vi "qp_find initial feasible solution.vi"(6 "tolerance":dbl=1e-05, 8 "error in (no error)":errorcluster, 11 "qp data in":T1) -> (0 "error out":errorcluster, 3 "qp data in":T1)   [LabVIEW 2014, in "NI_Gmath.lvlib"]
uses:
  NI_Gmath.lvlib
  qp_problem data.ctl
  A x Vector.vi
  Real A x B.vi
  Real Dot Product.vi
  Create Special Real Matrix.vi
  ones_1d.vi
  zeroes_1d.vi
  zeroes_2d.vi
  Matrix left divisionMM.vi
  NI_AALBase.lvlib
  NI_AALPro.lvlib
panel:
  out "Numeric":i32
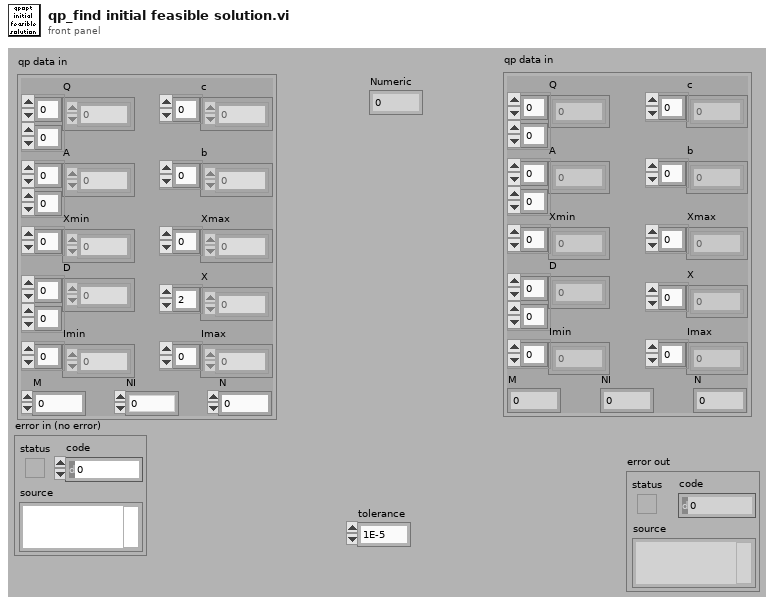
[diagram p1: front panel]
types:
  T1 = typedef "NI_Gmath.lvlib/qp_problem data.ctl" = cluster{"Q":dbl[][], "c":dbl[], "A":dbl[][], "b":dbl[], "Xmin":dbl[], "Xmax":dbl[], "M":i32, "N":i32, "D":dbl[][], "Imax":dbl[], "Imin":dbl[], "NI":i32, "X":dbl[]}
  T2 = enum32{"Identity", "Diagonal", "Toepliz", "Vandermonde", "Companion"}
  T3 = typedef "NI_Matrix.lvlib/RealMatrix.ctl" = dbl[][]
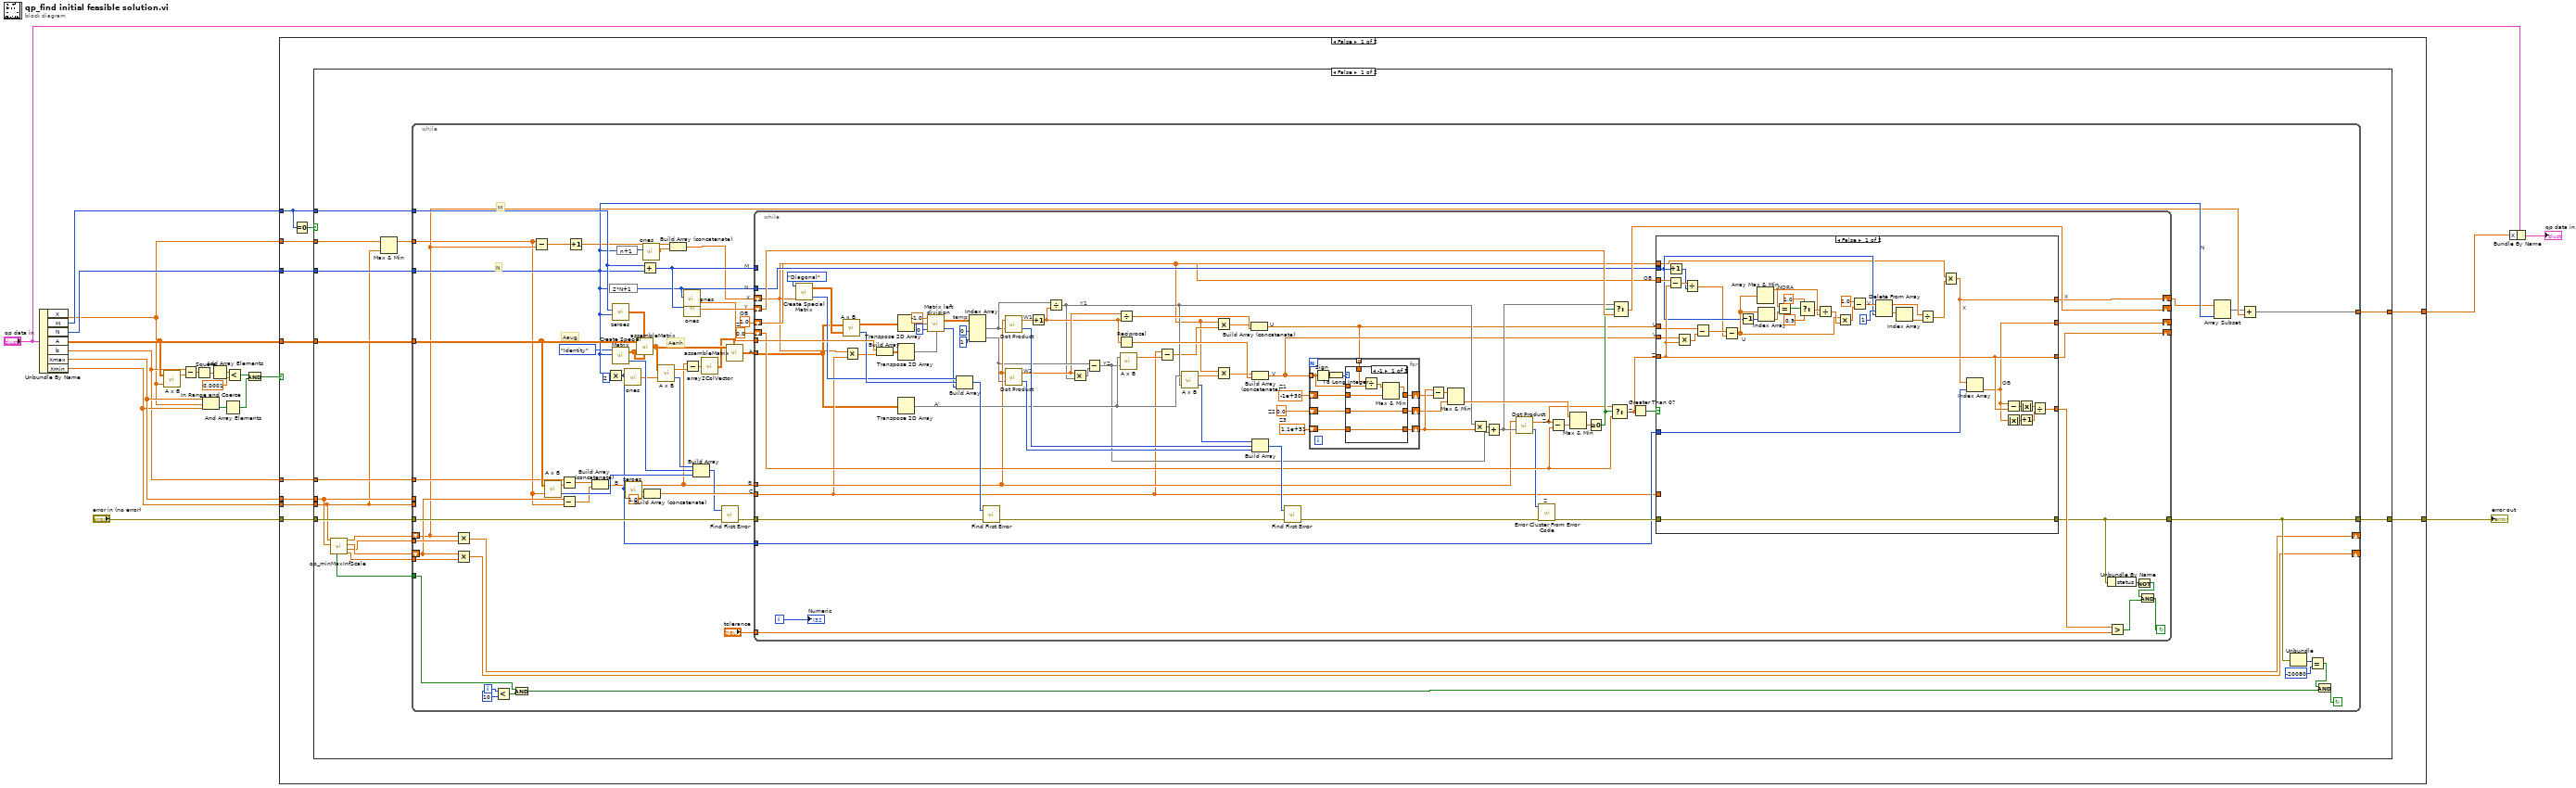
[diagram p0: block diagram]
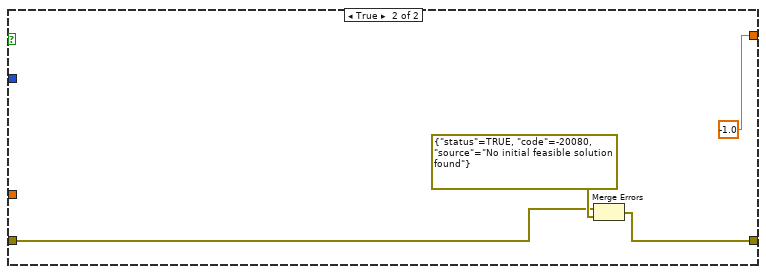
[diagram p2: hidden frame]
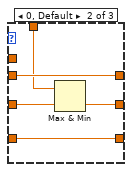
[diagram p3: hidden frame]
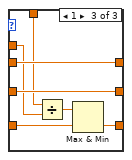
[diagram p4: hidden frame]
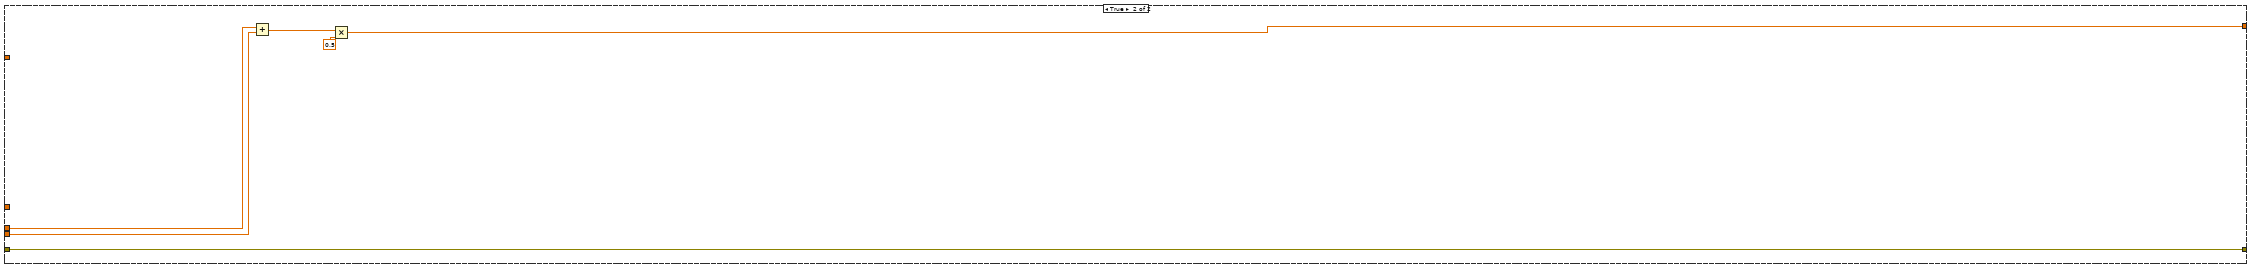
[diagram p5: hidden frame]
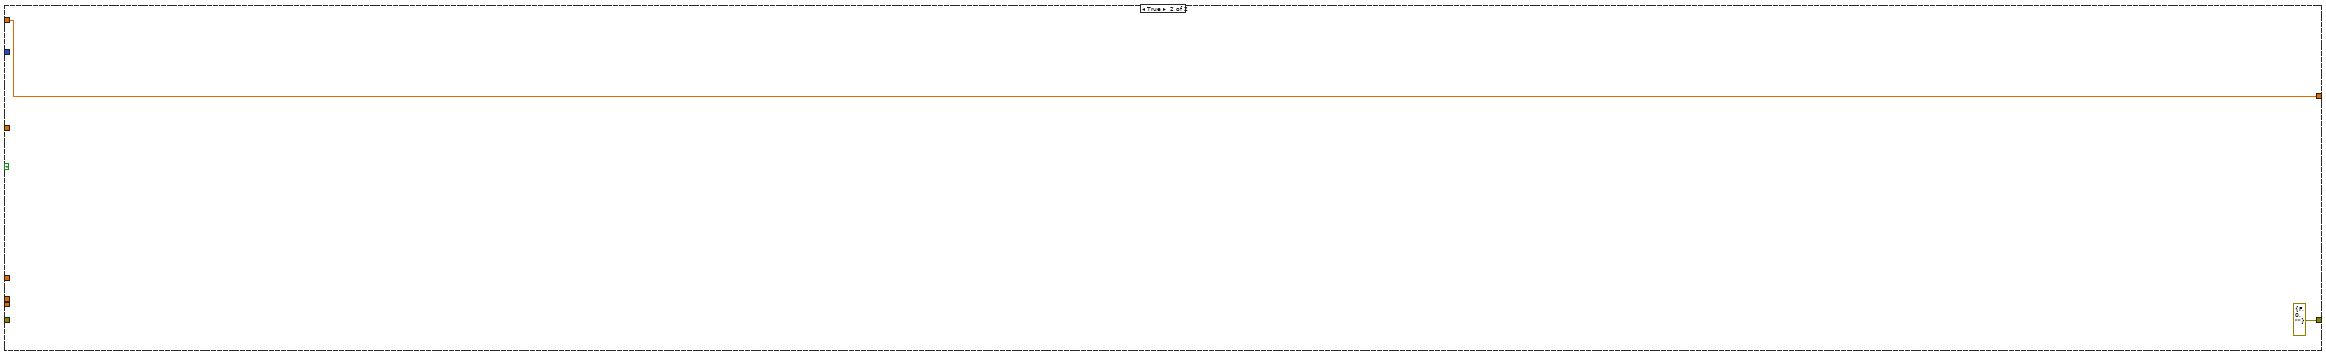
[diagram p6: hidden frame]
diagram:
  n1 = Unbundle By Name("qp data in") -> ("X"=w4:dbl[], "M"=w20:i32, "N"=w21:i32, "A"=w7:dbl[][], "b"=w6:dbl[], "Xmax"=w9:dbl[], "Xmin"=w8:dbl[])
  n2 = call-poly "A x B.vi"("Vector"=w4, "A"=w7) -> ("A x Vector"=w17:dbl[])  [unwired: 1 out]
  n3 = Subtract ("Subtract.vi")(x=w6, y=w17) -> (x-y=w16:dbl[])
  n4 = Square(x=w16) -> (x^2=w15:dbl[])
  n5 = In Range and Coerce(upper limit=w9, x=w4, lower limit=w8) -> (In Range?=w11:bool[])  [unwired: 1 out]
  n6 = Add Array Elements(numeric array=w15) -> (sum=w14:dbl)
  n7 = And Array Elements(Boolean array=w11) -> (logical AND=w10:bool)
  n8 = Less?(x=w14, y=0.0001) -> (x < y?=w12:bool)
  n9 = And(x=w12, y=w10) -> (x .and. y?=w5:bool)
  n10 = case shown="False" w5 {
    tunnel: w21 -> [w32 _]
    tunnel: w20 -> [w30 _]
    tunnel: [w29 errorcluster {"status"=FALSE, "code"=0, "source"=""} ("error in (no error)")] -> w19
    tunnel: "error in (no error)" -> [w28 _]
    tunnel: [w27 w267] -> w2
    tunnel: w4 -> [w26 w267]
    tunnel: w9 -> [w25 _]
    tunnel: w8 -> [w24 _]
    tunnel: w7 -> [w23 _]
    tunnel: w6 -> [w22 _]
    frame False {
      n11 = Equal To 0?(x=w30) -> (x = 0?=w31:bool)
      n12 = case shown="False" w31 {
        tunnel: [w47 w261] -> w27
        tunnel: w32 -> [w36 _]
        tunnel: w23 -> [w43 _]
        tunnel: w22 -> [w48 _]
        tunnel: w30 -> [w44 _]
        tunnel: [w46 w260] -> w29
        tunnel: w28 -> [w45 w260]
        tunnel: w24 -> [w35 w264]
        tunnel: w25 -> [w37 w265]
        tunnel: w26 -> [w33 _]
        frame False {
          n13 = call "qp_minMaxInfScale.vi"("Xmax"=w37, "Xmin"=w35) -> ("Xmax scale"=w39:dbl[], "Xmin scale"=w40:dbl[], "Xmax"=w41:dbl[], "Xmin"=w42:dbl[], "loop?"=w38:bool)  [unwired: 2 in]
          n14 = Max & Min(x=w33, y=w35) -> (max(x,y)=w34:dbl[])  [unwired: 1 out]
          n15 = while {
            tunnel: w48 -> [w90]
            tunnel: [w49] -> w47
            tunnel: [w96] -> w46
            tunnel: w45 -> [w108]
            tunnel: w44 -> [w107]
            tunnel: w43 -> [w106]
            tunnel: w36 -> [w105]
            tunnel: w34 -> [w51]
            shift-right: [w92] -> _
            shift-left: w42 -> [w88]
            shift-right: [w91] -> _
            shift-left: w41 -> [w89]
            tunnel: w40 -> [w94]
            tunnel: w39 -> [w93]
            tunnel: w38 -> [w101]
            tunnel: w37 -> [_]
            tunnel: w35 -> [_]
            i -> [w104]
            stop <- w100 continue-if-true
            w78 = 0.0  # Z
            w79 = 1.0  # OB
            # "Aaug"
            # "Aenh"
            # "M"
            # "N"
            # "N"
            # "Y"
            # "X"
            # "C"
            # "N"
            # "M"
            # "B"
            # "A"
            # "B"
            n16 = Multiply(x=w88, y=w94) -> (x*y=w92:dbl[])
            n17 = Multiply(x=w89, y=w93) -> (x*y=w91:dbl[])
            n18 = Less?(x=w104, y=10) -> (x < y?=w102:bool)
            n19 = And(x=w101, y=w102) -> (x .and. y?=w99:bool)
            n20 = Subtract(x=w51, y=w88) -> (x-y=w62:dbl[])
            n21 = call-poly "A x B.vi"("Vector"=w51, "A"=w106) -> ("error"=w87:i32, "A x Vector"=w84:dbl[])
            n22 = Subtract(x=w90, y=w84) -> (x-y=w63:dbl[])
            n23 = Subtract(x=w89, y=w51) -> (x-y=w60:dbl[])
            n24 = Increment(x=w62) -> (x+1=w61:dbl[])
            n25 = Build Array (concatenate)(w63, w60) -> (w56:dbl[])
            n26 = Multiply(x=w105, y=2) -> (x*y=w59:i32)
            n27 = expression code="2*N+1"(w105) -> (w52:i32)
            n28 = call-poly "zeroes.vi"("m"=w107, "n"=w105) -> ("ones"=w76:dbl[][])  [unwired: 6 in]
            n29 = call-poly "Create Special Matrix.vi"("matrix type"=T2."Identity", "matrix size"=w105) -> ("Special Matrix"=w83:T3, "error"=w86:i32)  [unwired: 3 in]
            n30 = expression code="n+1"(w105) -> (w65:i32)
            n31 = call-poly "ones.vi"("m"=w59) -> ("ones"=w77:dbl[])  [unwired: 7 in]
            n32 = call-poly "zeroes.vi"("m"=w59) -> ("ones"=w72:dbl[])  [unwired: 7 in]
            n33 = call "assembleMatrix.vi"("A"=w106, "B"=w76, "C"=w83, "D"=w83) -> ("ABCD"=w81:dbl[][])  [unwired: 1 in]
            n34 = Add(x=w107, y=w105) -> (x+y=w53:i32)
            n35 = call-poly "ones.vi"("m"=w65) -> ("ones"=w64:dbl[])  [unwired: 7 in]
            n36 = Build Array (concatenate)(w72, 1.0) -> (w70:dbl[])
            n37 = call-poly "A x B.vi"("Vector"=w77, "A"=w81) -> ("error"=w85:i32, "A x Vector"=w57:dbl[])
            n38 = Build Array (concatenate)(w61, w64) -> (w50:dbl[])
            n39 = call-poly "ones.vi"("m"=w52) -> ("ones"=w54:dbl[])  [unwired: 7 in]
            n40 = call-poly "ones.vi"("m"=w53) -> ("ones"=w75:dbl[])  [unwired: 7 in]
            n41 = Subtract(x=w56, y=w57) -> (x-y=w58:dbl[])
            n42 = Build Array(w85, w86, w87) -> (w68:i32[])
            n43 = call "array2ColVector.vi"("vector"=w58) -> ("col vector"=w55:dbl[][])
            n44 = call "Find First Error.vi"("error in (no error)"=w108, "error codes"=w68) -> ("error out"=w67:errorcluster)  [unwired: 2 in, 1 out]
            n45 = call "assembleMatrix.vi"("A"=w81, "B"=w55) -> ("ABCD"=w69:dbl[][])  [unwired: 3 in]
            n46 = while {
              tunnel: "tolerance" -> [w180]
              tunnel: w69 -> [w113]
              tunnel: w56 -> [w151]
              shift-right: [w156] -> _
              shift-left: w79 -> [w124]
              shift-right: [w155] -> _
              shift-left: w78 -> [w165]
              tunnel: w53 -> [_]
              tunnel: w52 -> [w157]
              tunnel: w70 -> [w118]
              shift-right: [w136] -> w74
              shift-left: w50 -> [w114]
              shift-right: [w162] -> _
              shift-left: w75 -> [w188]
              tunnel: w67 -> [w133]
              tunnel: [w125] -> w96
              tunnel: w59 -> [w123]
              tunnel: w54 -> [w189]
              i -> [w115]
              stop <- w126 continue-if-true
              w176 = 0.0  # Z2
              w174 = 1.1e+31  # Z3
              w175 = -1e+30  # Z1
              # "V"
              # "W2"
              # "W1"
              # "Y1"
              # "X"
              # "Z"
              # "V"
              # "U"
              # "OB"
              # "U"
              # "Z"
              # "Z4"
              # "Z"
              # "A'"
              # "Y2"
              # "temp"
              n47 = call-poly "Create Special Matrix.vi"("matrix type"=T2."Diagonal", "Input Vector1"=w114) -> ("Special Matrix"=w159:T3, "error"=w181:i32)  [unwired: 3 in]
              n48 = call-poly "A x B.vi"("B"=w159, "A"=w113) -> ("error"=w182:i32, "A x B"=w142:T3)
              n49 = Multiply(x=w114, y=w118) -> (x*y=w117:dbl[])
              n50 = Build Array(w189, w117) -> (w141:dbl[][])
              n51 = Transpose 2D Array(2D array=w142) -> (transposed array=w112:T3)
              n52 = Transpose 2D Array(2D array=w141) -> (transposed array=w110:dbl[][])
              n53 = Transpose 2D Array(2D array=w113) -> (transposed array=w177:dbl[][])
              n54 = call-poly "Matrix left division.vi"("A"=w110, "number of iterations"=0, "B"=w112, "SVD relative tolerance"=-1.0) -> ("error"=w116:i32, "B\\A"=w135:dbl[][])
              n55 = Build Array(w181, w182, w116) -> (w183:i32[])
              n56 = Index Array(array=w135, index (col) #1=0, index (col) #2=1) -> (element #1=w140:dbl[], element #2=w148:dbl[])  [unwired: 2 in]
              n57 = call "Find First Error.vi"("error in (no error)"=w133, "error codes"=w183) -> ("error out"=w134:errorcluster)  [unwired: 2 in, 1 out]
              n58 = call-poly "Dot Product.vi"("Y Vector"=w140, "X Vector"=w151) -> ("error"=w185:i32, "X * Y"=w154:dbl)
              n59 = call-poly "Dot Product.vi"("Y Vector"=w148, "X Vector"=w151) -> ("error"=w186:i32, "X * Y"=w147:dbl)
              n60 = Increment(x=w154) -> (x+1=w145:dbl)
              n61 = Divide(x=w140, y=w145) -> (x/y=w139:dbl[])
              n62 = Multiply(x=w147, y=w139) -> (x*y=w152:dbl[])
              n63 = Subtract(x=w148, y=w152) -> (x-y=w153:dbl[])
              n64 = Divide(x=w147, y=w145) -> (x/y=w146:dbl)
              n65 = Reciprocal(x=w145) -> (1/x=w144:dbl)
              n66 = call-poly "A x B.vi"("Vector"=w153, "A"=w177) -> ("A x Vector"=w178:dbl[])  [unwired: 1 out]
              n67 = Subtract(x=w118, y=w178) -> (x-y=w122:dbl[])
              n68 = call-poly "A x B.vi"("Vector"=w139, "A"=w177) -> ("error"=w184:i32, "A x Vector"=w120:dbl[])
              n69 = Multiply(x=w114, y=w122) -> (x*y=w121:dbl[])
              n70 = Multiply(x=w114, y=w120) -> (x*y=w119:dbl[])
              n71 = Build Array (concatenate)(w121, w146) -> (w137:dbl[])
              n72 = Build Array (concatenate)(w119, w144) -> (w138:dbl[])
              n73 = Build Array(w184, w185, w186) -> (w187:i32[])
              n74 = call "Find First Error.vi"("error in (no error)"=w134, "error codes"=w187) -> ("error out"=w131:errorcluster)  [unwired: 2 in, 1 out]
              n75 = for {
                tunnel: w138 -> [w234] mode=indexing
                shift-right: [w231] -> w171
                shift-left: w175 -> [w238]
                shift-right: [w233] -> w169
                shift-left: w176 -> [w237]
                shift-right: [w232] -> w172
                shift-left: w174 -> [w236]
                tunnel: w137 -> [w235] mode=indexing
                n76 = Sign(1:w234) -> (0:w240:dbl)
                n77 = To Long Integer(number=w240) -> (32bit integer=w239:i32)
                n78 = case shown="-1" w239 {
                  tunnel: w238 -> [w244 w251 w259]
                  tunnel: w237 -> [w243 w252 w258]
                  tunnel: w236 -> [w242 w250 w254]
                  tunnel: w235 -> [w247 w249 w257]
                  tunnel: w234 -> [w246 _ w256]
                  tunnel: [w243 w248 w258] -> w233
                  tunnel: [w242 w250 w253] -> w232
                  tunnel: [w241 w251 w259] -> w231
                  frame -1 {
                    n79 = Divide(x=w247, y=w246) -> (x/y=w245:dbl)
                    n80 = Max & Min(x=w245, y=w244) -> (max(x,y)=w241:dbl)  [unwired: 1 out]
                  }
                  frame 0, Default {
                    n81 = Max & Min(x=w249, y=w252) -> (min(x,y)=w248:dbl)  [unwired: 1 out]
                  }
                  frame 1 {
                    n82 = Divide(x=w257, y=w256) -> (x/y=w255:dbl)
                    n83 = Max & Min(x=w255, y=w254) -> (min(x,y)=w253:dbl)  [unwired: 1 out]
                  }
                }
              }
              n84 = Subtract(x=w172, y=w171) -> (x-y=w170:dbl)
              n85 = Max & Min(x=w170, y=w169) -> (min(x,y)=w168:dbl)  [unwired: 1 out]
              n86 = Multiply(x=w139, y=w172) -> (x*y=w173:dbl[])
              n87 = Add(x=w173, y=w153) -> (x+y=w163:dbl[])
              n88 = call-poly "Dot Product.vi"("Y Vector"=w163, "X Vector"=w151) -> ("error"=w132:i32, "X * Y"=w143:dbl)
              n89 = call "Error Cluster From Error Code.vi"("error in (no error)"=w131, "error code (0)"=w132) -> ("error out"=w130:errorcluster)  [unwired: 7 in]
              n90 = Subtract(x=w143, y=w165) -> (x-y=w167:dbl)
              n91 = Max & Min(x=w168, y=w167) -> (min(x,y)=w166:dbl)  [unwired: 1 out]
              n92 = Greater Or Equal To 0?(x=w166) -> (x >= 0?=w164:bool)
              n93 = Select(t=w143, s=w164, f=w165) -> (s? t:f=w158:dbl)
              n94 = Select(t=w163, s=w164, f=w188) -> (s? t:f=w162:dbl[])
              n95 = Greater Than 0?(x=w158) -> (x > 0?=w161:bool)
              n96 = case shown="False" w161 {
                tunnel: [w207 -1.0 ("GoGo")] -> w160
                tunnel: w137 -> [w224 _]
                tunnel: w138 -> [w225 _]
                tunnel: w158 -> [w226 _]
                tunnel: w124 -> [w222 _]
                tunnel: w157 -> [w199 _]
                tunnel: [w191 _] -> w136
                tunnel: w118 -> [_ _]
                tunnel: [w194 _] -> w156
                tunnel: [w226 _] -> w155
                tunnel: w130 -> [w190 w228]
                tunnel: [w190 w227] -> w125
                tunnel: w123 -> [w195 _]
                tunnel: w114 -> [w192 _]
                frame False {
                  # "X"
                  # "OB"
                  # "V"
                  # "U"
                  # "NORA"
                  n97 = Subtract(x=w222, y=w226) -> (x-y=w221:dbl)
                  n98 = Increment(x=w199) -> (x+1=w220:i32)
                  n99 = Multiply(x=w225, y=w226) -> (x*y=w223:dbl[])
                  n100 = Divide(x=w221, y=w220) -> (x/y=w197:dbl)
                  n101 = Subtract(x=w224, y=w223) -> (x-y=w218:dbl[])
                  n102 = Subtract(x=w218, y=w197) -> (x-y=w203:dbl[])
                  n103 = Decrement(x=w199) -> (x-1=w202:i32)
                  n104 = Array Max & Min(array=w203) -> (max value=w213:dbl)  [unwired: 3 out]
                  n105 = Index Array(array=w203, index=w202) -> (element=w219:dbl)
                  n106 = Equal?(x=w213, y=w219) -> (x = y?=w217:bool)
                  n107 = Select(t=1.0, s=w217, f=0.9) -> (s? t:f=w214:dbl)
                  n108 = Divide(x=w214, y=w213) -> (x/y=w212:dbl)
                  n109 = Multiply(x=w203, y=w212) -> (x*y=w211:dbl[])
                  n110 = Subtract(x=1.0, y=w211) -> (x-y=w201:dbl[])
                  n111 = Delete From Array(array=w201, length=1, index=w199) -> (deleted portion=w205:dbl[], array with subset deleted=w200:dbl[])
                  n112 = Index Array(array=w205) -> (element=w204:dbl)  [unwired: 1 in]
                  n113 = Divide(x=w200, y=w204) -> (x/y=w193:dbl[])
                  n114 = Multiply(x=w192, y=w193) -> (x*y=w191:dbl[])
                  n115 = Index Array(array=w191, index=w195) -> (element=w194:dbl)
                  n116 = Subtract(x=w194, y=w226) -> (x-y=w210:dbl)
                  n117 = Absolute Value(x=w194) -> (abs(x)=w209:dbl)
                  n118 = Absolute Value(x=w210) -> (abs(x)=w198:dbl)
                  n119 = Increment(x=w209) -> (x+1=w208:dbl)
                  n120 = Divide(x=w198, y=w208) -> (x/y=w207:dbl)
                }
                frame True {
                  n121 = Merge Errors(w228, errorcluster {"status"=TRUE, "code"=-20080, "source"="No initial feasible solution found"} ("error out")) -> (w227:errorcluster)
                }
              }
              n122 = Unbundle By Name(w125) -> ("status"=w129:bool)
              n123 = Greater?(x=w160, y=w180) -> (0:w127:bool)
              n124 = Not(x=w129) -> (.not. x?=w128:bool)
              n125 = And(x=w128, y=w127) -> (x .and. y?=w126:bool)
              "Numeric" <- w115
            }
            n126 = Array Subset(array=w74, length=w105) -> (w73:dbl[])  [unwired: 1 in]
            n127 = Add(x=w73, y=w88) -> (x+y=w49:dbl[])
            n128 = Unbundle(w96) -> ("code"=w97:i32)  [unwired: 2 out]
            n129 = Equal?(x=w97, y=-20080) -> (x = y?=w95:bool)
            n130 = And(x=w95, y=w99) -> (x .and. y?=w100:bool)
          }
        }
        frame True {
          n131 = Add(x=w265, y=w264) -> (x+y=w263:dbl[])
          n132 = Multiply(x=w263, y=0.5) -> (x*y=w261:dbl[])
        }
      }
    }
    frame True {
    }
  }
  "error out" <- w19
  n133 = Bundle By Name(cluster="qp data in", "X"=w2) -> (→"qp data in":T1)
